vi "VerifyTargetIP.vi"(8 "error in (no error)":errorcluster, 11 "Target":string) -> (0 "error out":errorcluster, 3 "IP Address String out":string)   [LabVIEW 2017, in "Shared Variables CD 2.0 Configuration.lvlib"]
uses:
  Shared Variables CD 2.0 Configuration.lvlib
  <vilib>/Utility/error.llb/Error Cluster From Error Code.vi
  <vilib>/ErrorRing/Error Ring.xnode
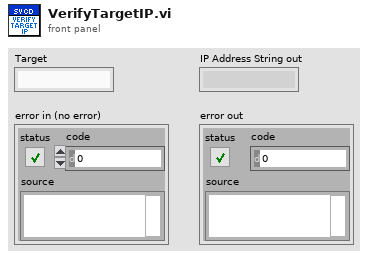
[diagram p1: front panel]
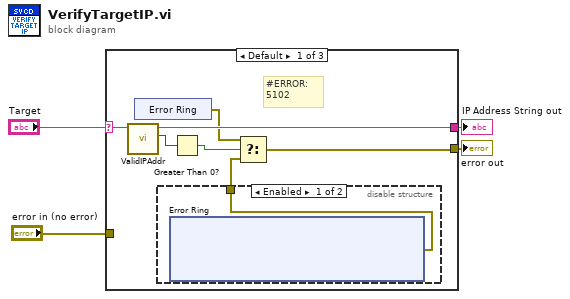
[diagram p0: block diagram]
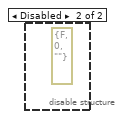
[diagram p2: hidden frame]
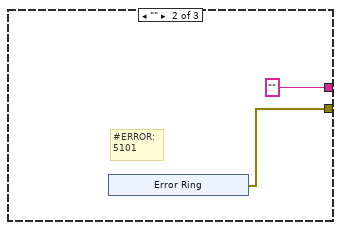
[diagram p3: hidden frame]
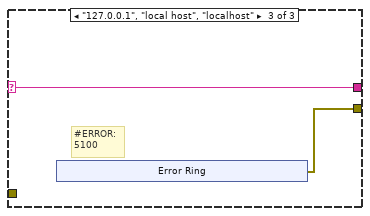
[diagram p4: hidden frame]
diagram:
  n1 = case shown="Default" "Target" {
    selector: "Target" -> [w11 _ w22]
    tunnel: "error in (no error)" -> [_ _ _]
    tunnel: [w6 w15 w23] -> w3
    tunnel: [w10 "" w22] -> w4
    frame Default {
      # "#ERROR:\n5102"
      n2 = call "ValidIPAddr.vi"("IP Address String"=w11) -> ("return type"=w9:i32, "IP Address String out"=w10:string)  [unwired: 8 in, 1 out]
      n3 = xnode "Error Ring"() -> ("error out"=w5:errorcluster)
      n4 = disable-structure shown="Enabled" {
        disable-tunnel: [w13 _] -> w7
        frame Enabled {
          n5 = xnode "Error Ring"() -> ("error out"=w13:errorcluster)
        }
        frame Disabled {
          (unwired) errorcluster {"status"=FALSE, "code"=0, "source"=""} ("error out")
        }
      }
      n6 = Greater Than 0?(x=w9) -> (x > 0?=w8:bool)
      n7 = Select(t=w5, s=w8, f=w7) -> (s? t:f=w6:errorcluster)
    }
    frame "" {
      # "#ERROR:\n5101"
      n8 = xnode "Error Ring"() -> ("error out"=w15:errorcluster)
    }
    frame "127.0.0.1", "local host", "localhost" {
      # "#ERROR:\n5100"
      n9 = xnode "Error Ring"() -> ("error out"=w23:errorcluster)
    }
  }
  "IP Address String out" <- w4
  "error out" <- w3
